vi "String To Array.vi"(0 "String":string, 5 "delimiter (Tab)":string, 11 "error in (no error)":errorcluster) -> (4 "1DArray":string[](array[string]), 15 "error out":errorcluster)   [LabVIEW 2021, in "CustomSortPath.lvlib"]
doc: "Gets the string and delimiter as input and converts the string to 1D string array."
uses:
  CustomSortPath.lvlib
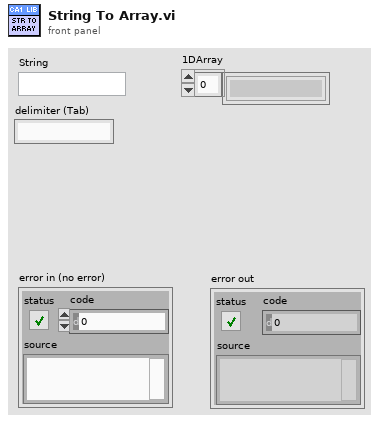
[diagram p1: front panel]
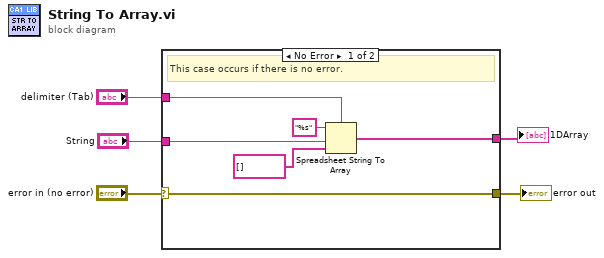
[diagram p0: block diagram]
diagram:
  n1 = case shown="No Error" "error in (no error)" {
    selector: "error in (no error)" -> [w9 w12]
    tunnel: [w9 w12] -> w4
    tunnel: [w8 _] -> w3
    tunnel: "delimiter (Tab)" -> [w7 _]
    tunnel: "String" -> [w6 _]
    frame No Error {
      # "This case occurs if there is no error."
      n2 = Spreadsheet String To Array(delimiter (Tab)=w7, format string="%s", spreadsheet string=w6, array type (2D Dbl)=string[] []) -> (array=w8:string[])
    }
    frame Error {
      # "This case occurs if there is any error."
    }
  }
  "error out" <- w4
  "1DArray" <- w3
